vi "ScanlistFormats.vi"(6 "FirstMeasNmInd":i32, 8 "ErrorIn(No Error)":errorcluster caption="entrée d'erreur (pas d'erreur)", 9 "IndCourbe":i64, 10 "DatNmSuffix":string, 11 "DatNmArr":string[](array[string])) -> (0 "Err Out":errorcluster caption="sortie d'erreur", 2 "VarParList":string[](array[string]), 3 "ScanList":string[](array[string]))   [LabVIEW 2019]
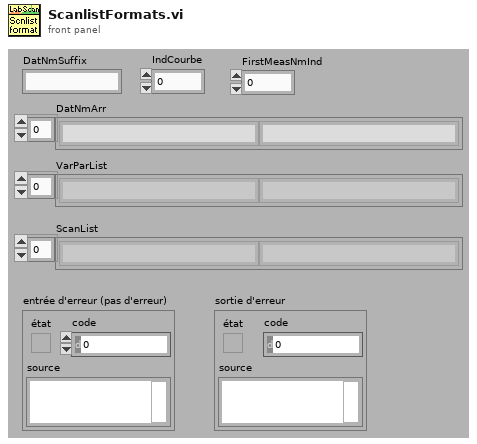
[diagram p1: front panel]
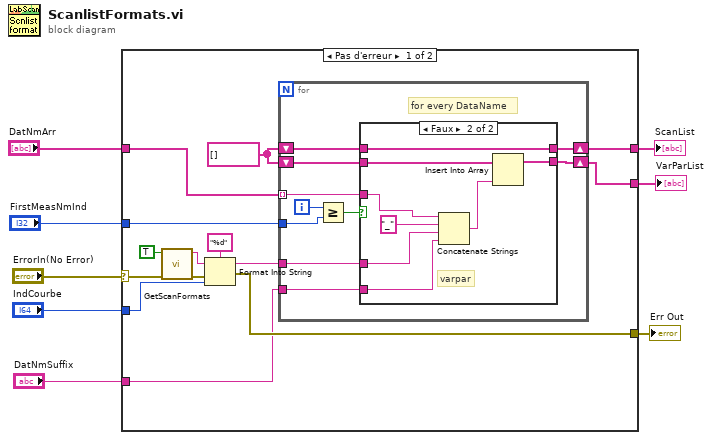
[diagram p0: block diagram]
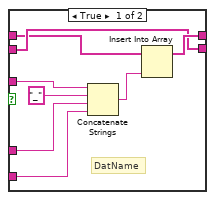
[diagram p2: hidden frame]
diagram:
  n1 = case shown="Pas d'erreur" "ErrorIn(No Error)" {
    selector: "ErrorIn(No Error)" -> [w18 w49]
    tunnel: [w16 w49] -> w7
    tunnel: "IndCourbe" -> [w19 _]
    tunnel: "DatNmSuffix" -> [w11 _]
    tunnel: "DatNmArr" -> [w14 _]
    tunnel: [w10 _] -> w3
    tunnel: "FirstMeasNmInd" -> [w13 _]
    tunnel: [w9 _] -> w1
    frame No Error {
      w15 = string[] []
      n2 = call "GetScanFormats.vi"("ErrorIn(No Error)"=w18, "Scan(T)"=TRUE) -> ("sortie d'erreur"=w17:errorcluster, "Prefixe"=w20:string)  [unwired: 7 in, 1 out]
      n3 = Format Into String(format string="%d" ("chaîne de format"), initial string=w20, error in=w17, w19) -> (resulting string=w12:string, error out=w16:errorcluster)
      n4 = for {
        tunnel: w12 -> [w30]
        tunnel: w14 -> [w31] mode=indexing
        shift-right: [w23] -> w9
        shift-left: w15 -> [w32]
        tunnel: w13 -> [w29]
        shift-right: [w25] -> w10
        shift-left: w15 -> [w26]
        tunnel: w11 -> [w24]
        i -> [w28]
        # "for every DataName"
        n5 = Greater Or Equal?(x=w28, y=w29) -> (x >= y?=w27:bool)
        n6 = case shown="Faux" w27 {
          tunnel: w32 -> [w33 w43]
          tunnel: [w40 w43] -> w23
          tunnel: w31 -> [w39 w41]
          tunnel: w30 -> [w38 w48]
          tunnel: w26 -> [w35 w45]
          tunnel: [w35 w44] -> w25
          tunnel: w24 -> [w34 w42]
          frame True {
            # "DatName"
            n7 = Concatenate Strings(w39, "_" ("chaîne"), w38, w34) -> (w37:string)
            n8 = Insert Into Array(array=w33, new element=w37) -> (w40:string[])  [unwired: 1 in]
          }
          frame False {
            # "varpar"
            n9 = Concatenate Strings(w41, "_" ("chaîne"), w48, w42) -> (w47:string)
            n10 = Insert Into Array(array=w45, new element=w47) -> (w44:string[])  [unwired: 1 in]
          }
        }
      }
    }
    frame Error {
    }
  }
  "Err Out" <- w7
  "VarParList" <- w3
  "ScanList" <- w1
